vi "KB-DataCollect.vi"(7 "Start Time":string, 8 "Porduct Color":string, 9 "Resultstring":string, 10 "Barcode":string, 11 "Data Result":string[][](array[string])=[["Null", "Null", "Null", "Null", "Null", "Null", "Null", "Null", "Null", "Null", "Null", "Null", "Null", "Null", "Null", "Null", "Null", "Null", "Null", "Null", "Null", "Null", "Null", "Null", "Null", "Null", "Null", "Null", "Null", "Null", "Null", "Null", "Null"], ["Null", "Null", "Null", "Null", "Null", "Null", "Null", "Null", "Null", "Null", "Null", "Null", "Null", "Null", "Null", "Null", "Null", "Null", "Null", "Null", "Null", "Null", "Null", "Null", "Null", "Null", "Null", "Null", "Null", "Null", "Null", "Null", "Null"], ["Null", "Null", "Null", "Null", "Null", "Null", "Null", "Null", "Null", "Null", "Null", "Null", "Null", "Null", "Null", "Null", "Null", "Null", "Null", "Null", "Null", "Null", "Null", "Null", "Null", "Null", "Null", "Null", "Null", "Null", "Null", "Null", "Null"], ["Null", "Null", "Null", "Null", "Null", "Null", "Null", "Null", "Null", "Null", "Null", "Null", "Null", "Null", "Null", "Null", "Null", "Null", "Null", "Null", "Null", "Null", "Null", "Null", "Null", "Null", "Null", "Null", "Null", "Null", "Null", "Null", "Null"], ["Null", "Null", "Null", "Null", "Null", "Null", "Null", "Null", "Null", "Null", "Null", "Null", "Null", "Null", "Null", "Null", "Null", "Null", "Null", "Null", "Null", "Null", "Null", "Null", "Null", "Null", "Null", "Null", "Null", "Null", "Null", "Null", "Null"], ["Null", "Null", "Null", "Null", "Null", "Null", "Null", "Null", "Null", "Null", "Null", "Null", "Null", "Null", "Null", "Null", "Null", "Null", "Null", "Null", "Null", "Null", "Null", "Null", "Null", "Null", "Null", "Null", "Null", "Null", "Null", "Null", "Null"], ["Null", "Null", "Null", "Null", "Null", "Null", "Null", "Null", "Null", "Null", "Null", "Null", "Null", "Null", "Null", "Null", "Null", "Null", "Null", "Null", "Null", "Null", "Null", "Null", "Null", "Null", "Null", "Null", "Null", "Null", "Null", "Null", "Null"]]) -> (3 "Result":string[](array[string]))   [LabVIEW 2015]
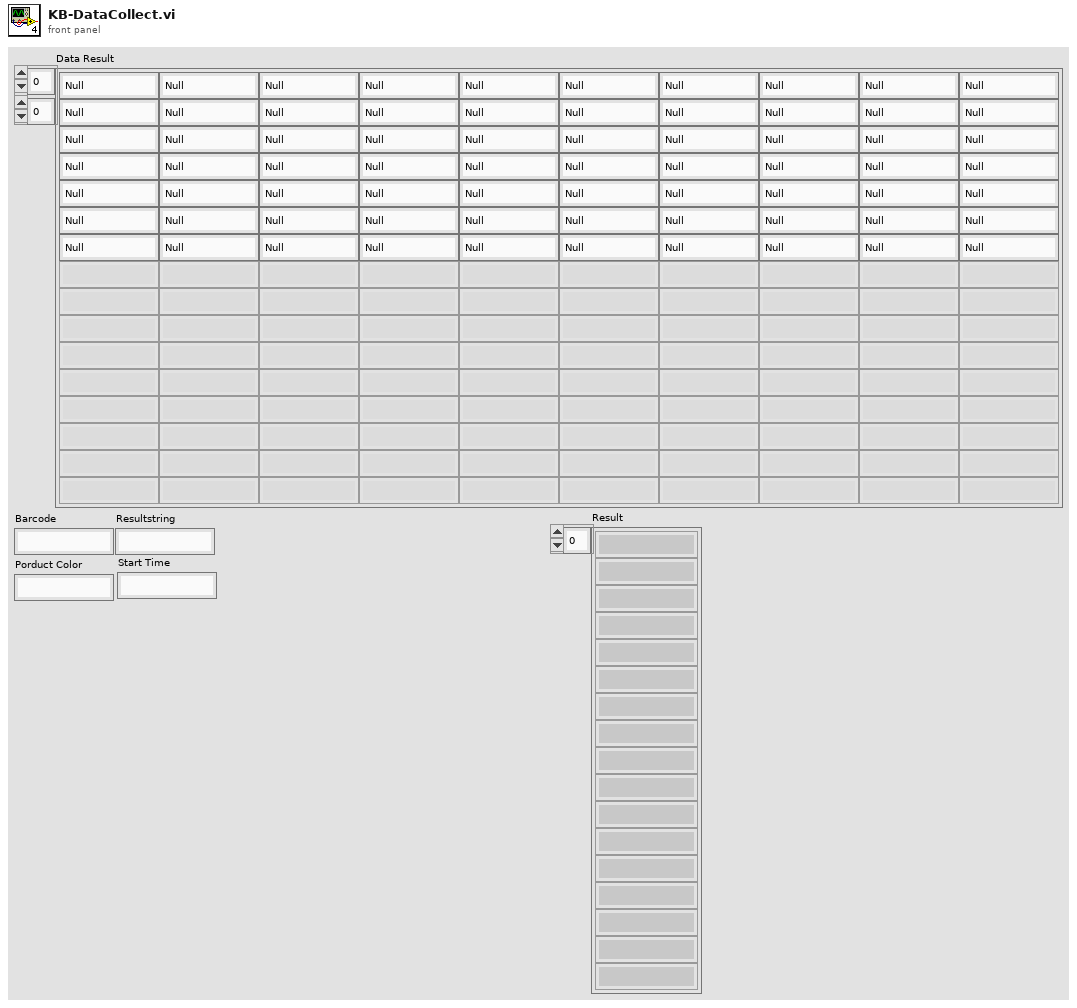
[diagram p1: front panel]
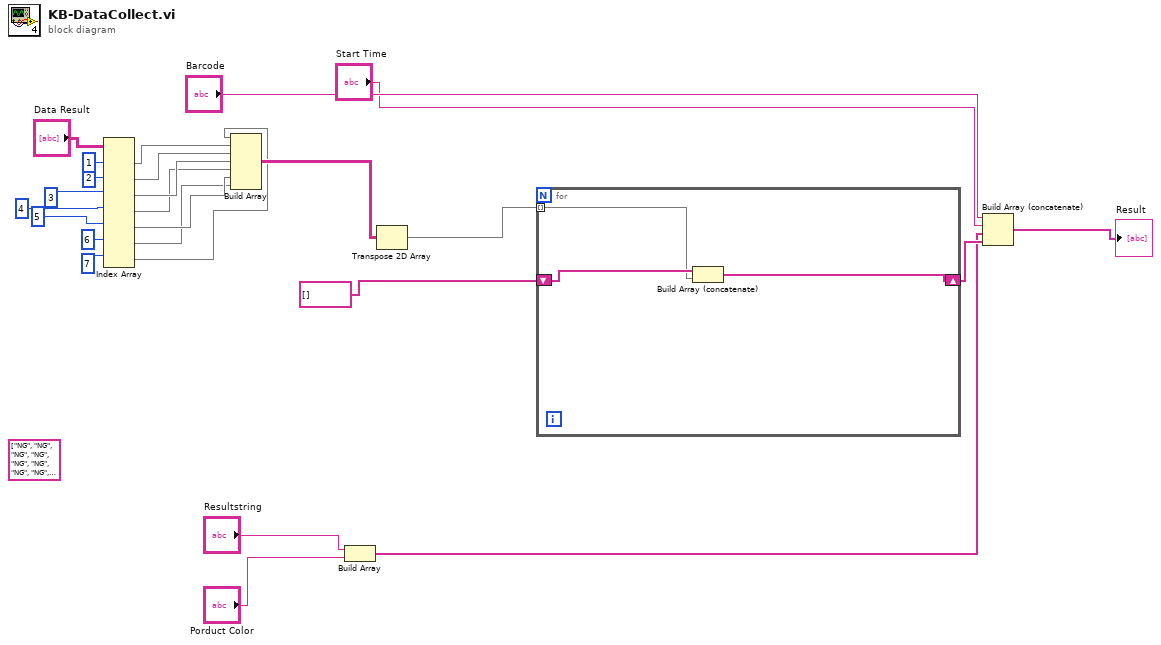
[diagram p0: block diagram]
diagram:
  (unwired) string[][] [["NG", "NG", "NG", "NG", "NG", "NG", "NG", "NG", "NG", "NG", "NG", "NG", "NG", "NG", "NG", "NG", "NG", "NG", "NG", "NG", "NG", "NG", "NG", "NG", "NG", "NG", "NG", "NG", "NG", "NG", "NG"], ["1", "1", "1", "1", "1", "1", "1", "1", "1", "1", "1", "1", "1", "1", "1", "1", "1", "1", "1", "1", "1", "1", "1", "1", "1", "1", "1", "1", "1", "1", "1"], ["2", "2", "2", "2", "2", "2", "2", "2", "2", "2", "2", "2", "2", "2", "2", "2", "2", "2", "2", "2", "2", "2", "2", "2", "2", "2", "2", "2", "2", "2", "2"], ["3", "3", "3", "3", "3", "3", "3", "3", "3", "3", "3", "3", "3", "3", "3", "3", "3", "3", "3", "3", "3", "3", "3", "3", "3", "3", "3", "3", "3", "3", "3"], ["0.126   mm", "0.033   mm", "0.079   mm", "0.009   mm", "0.058   mm", "0.077   mm", "0.035   mm", "0.026   mm", "0.026   mm", "0.015   mm", "0.010   mm", "0.060   mm", "0.233   mm", "0.033   mm", "0.028   mm", "0.047   mm", "0.065   mm", "0.022   mm", "0.104   mm", "0.056   mm", "0.040   mm", "0.032   mm", "0.073   mm", "0.377   mm", "0.084   mm", "0.105   mm", "0.045   mm", "0.019   mm", "0.027   mm", "0.084   mm", "0.055   mm"], ["金色", "金色", "金色", "金色", "金色", "金色", "金色", "金色", "金色", "金色", "金色", "金色", "银色", "银色", "银色", "银色", "金色", "金色", "金色", "金色", "金色", "银色", "银色", "银色", "银色", "金色", "银色", "银色", "银色", "银色", "金色"], ["无漏装", "无漏装", "无漏装", "无漏装", "无漏装", "无漏装", "无漏装", "无漏装", "无漏装", "无漏装", "无漏装", "无漏装", "无漏装", "无漏装", "无漏装", "无漏装", "无漏装", "无漏装", "无漏装", "无漏装", "无漏装", "无漏装", "无漏装", "无漏装", "无漏装", "无漏装", "无漏装", "无漏装", "无漏装", "无漏装", "无漏装"]] ("Data Result")
  n1 = Index Array(array="Data Result", index (row) #1=1 ("索引 (行)"), index (row) #2=2 ("索引 (行)"), index (row) #3=3 ("禁用的索引 (列)"), index (row) #4=4 ("索引 (行)"), index (row) #5=5 ("索引 (行)"), index (row) #6=6 ("索引 (行)"), index (row) #7=7 ("禁用的索引 (列)")) -> (element #1=w17:string[], element #2=w16:string[], element #3=w15:string[], element #4=w14:string[], element #5=w13:string[], element #6=w12:string[], element #7=w1:string[])  [unwired: 7 in]
  n2 = Build Array(w1, w17, w16, w15, w14, w13, w12) -> (w11:string[][])
  n3 = Build Array("Resultstring", "Porduct Color") -> (w4:string[])
  n4 = Transpose 2D Array(2D array=w11) -> (transposed array=w24:string[][])
  n5 = for {
    tunnel: w24 -> [w27] mode=indexing
    shift-right: [w26] -> w8
    shift-left: string[] [] -> [w28]
    n6 = Build Array (concatenate)(w28, w27) -> (w26:string[])
  }
  n7 = Build Array (concatenate)("Barcode", "Start Time", w4, w8) -> (→"Result":string[])
